vi "CDMA_TxPluseShaping.vi"(8 "error in (no error)":errorcluster caption="错误输入（无错误）", 9 "sampleRate":dbl, 10 "sc_data":cdb[](array[numeric]), 11 "Path":path) -> (0 "error out":errorcluster caption="错误输出", 2 "tx_data":cdb[](array[numeric]), 3 "Path Out":path)   [LabVIEW 2015]
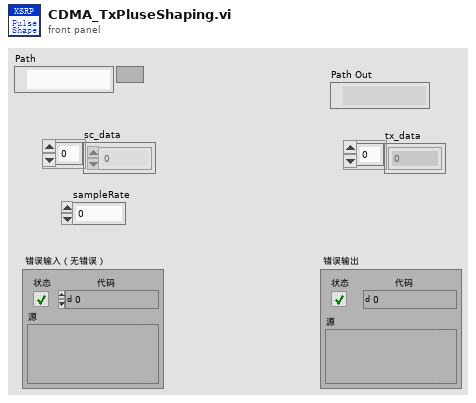
[diagram p1: front panel]
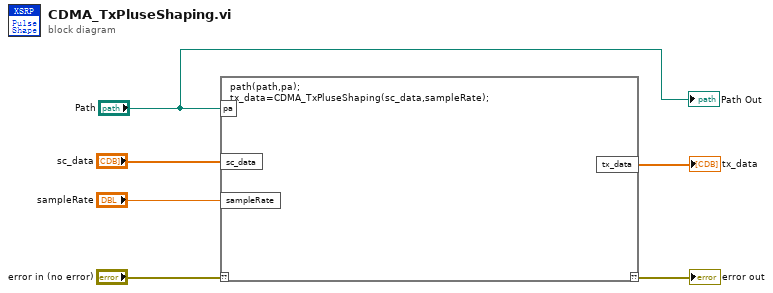
[diagram p0: block diagram]
diagram:
  n1 = script code="path(path,pa);\ntx_data=CDMA_TxPluseShaping(sc_data,sampleRate);"("??"="error in (no error)", "pa"="Path", "sc_data"="sc_data", "sampleRate"="sampleRate") -> ("??"=→"error out":errorcluster, "tx_data"=→"tx_data":cdb[])
  "Path Out" <- "Path"
